vi "Set HighLimit.vi"(8 "error in":errorcluster, 10 "Value":refnum<class "Value.lvclass">, 11 "Object Type in":refnum<class "Object Type Base.lvclass">) -> (0 "error out":errorcluster, 3 "Object Type out":refnum<class "Object Type Base.lvclass">)   [LabVIEW 2024, in "Electronic Datasheet.lvlib" / "Object Type Base.lvclass"]
uses:
  Object Type Base.lvclass
  Value/Value.lvclass
  Object Type Base.lvclass/Object Type Base.ctl
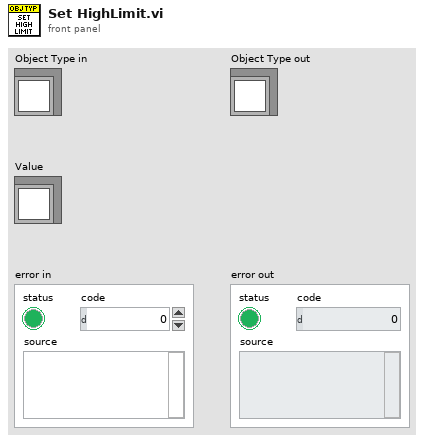
[diagram p1: front panel]
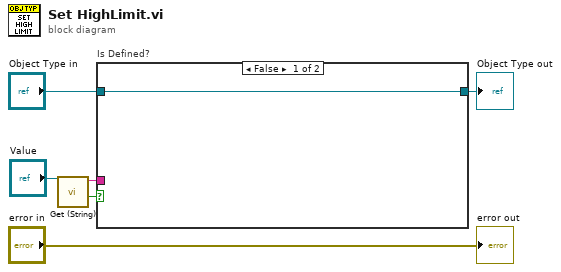
[diagram p0: block diagram]
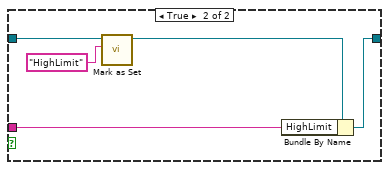
[diagram p2: hidden frame]
diagram:
  n1 = call "Get (String).vi"("Value in"="Value") -> ("Defined?"=w2:bool, "Value"=w4:string)  [unwired: 8 in, 1 out]
  n2 = case "Is Defined?" shown="False" w2 {
    tunnel: [w7 w12] -> w6
    tunnel: w4 -> [_ w11]
    tunnel: "Object Type in" -> [w7 w10]
    frame False {
    }
    frame True {
      n3 = call "Mark as Set.vi"("Field name"="HighLimit", "Object Type in"=w10) -> ("Object Type out"=w9:refnum<class "Object Type Base.lvclass">)  [unwired: 9 in]
      n4 = Bundle By Name(cluster=w9, "HighLimit"=w11) -> (w12:refnum<class "Object Type Base.lvclass">)
    }
  }
  "Object Type out" <- w6
  "error out" <- "error in"
